vi "sequencerStayInState.vi"(4 "stateBefore":T1) -> (1 "cmdByHost":T1)   [LabVIEW 2014]
uses:
  sequencerState.ctl
  <vilib>/rvi/Emulation/niFpgaGetClockAttributes.vi
  <vilib>/rvi/Emulation/niFpgaSctlEmulationGetInTimedLoop.vi
  <vilib>/rvi/Emulation/niFpgaEmulationReportErrorSimple.vi
  sequencerGlobVars.vi
  <vilib>/rvi/Emulation/niFpgaCriticalErrorInLSC.vi
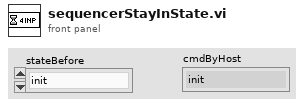
[diagram p1: front panel]
types:
  T1 = typedef "sequencerState.ctl" = enum16{"init", "idle", "writeGlobVars", "measureOffset", "measureTrack", "measComplete", "error"}
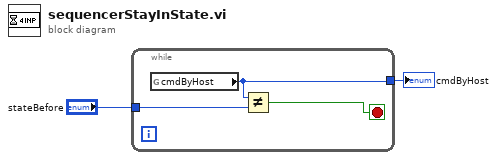
[diagram p0: block diagram]
diagram:
  n1 = while {
    tunnel: "stateBefore" -> [w5]
    tunnel: [w3] -> w1
    stop <- w4 stop-if-true
    n2 = global read "sequencerGlobVars.vi" "cmdByHost"() -> (w3:T1)
    n3 = Not Equal?(x=w3, y=w5) -> (x != y?=w4:bool)
  }
  "cmdByHost" <- w1
